vi "cwave_herbert.vi"(5 "Timing input":path=path "D:/Herbert/MeTimingDLL_test/bin/Release/MOTConf.csv", 8 "error in (no error)":errorcluster, 10 "Loop number":i16, 11 "Update rate (kHz)":i32=20) -> (0 "error out":errorcluster)   [LabVIEW 2009]
uses:
  dll.dll
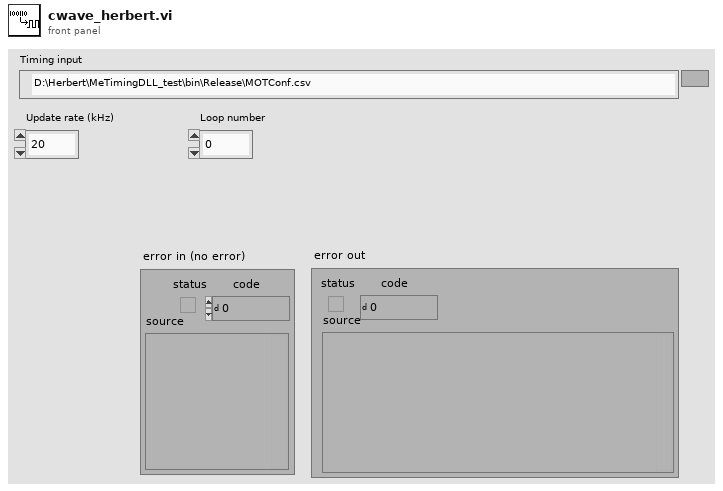
[diagram p1: front panel]
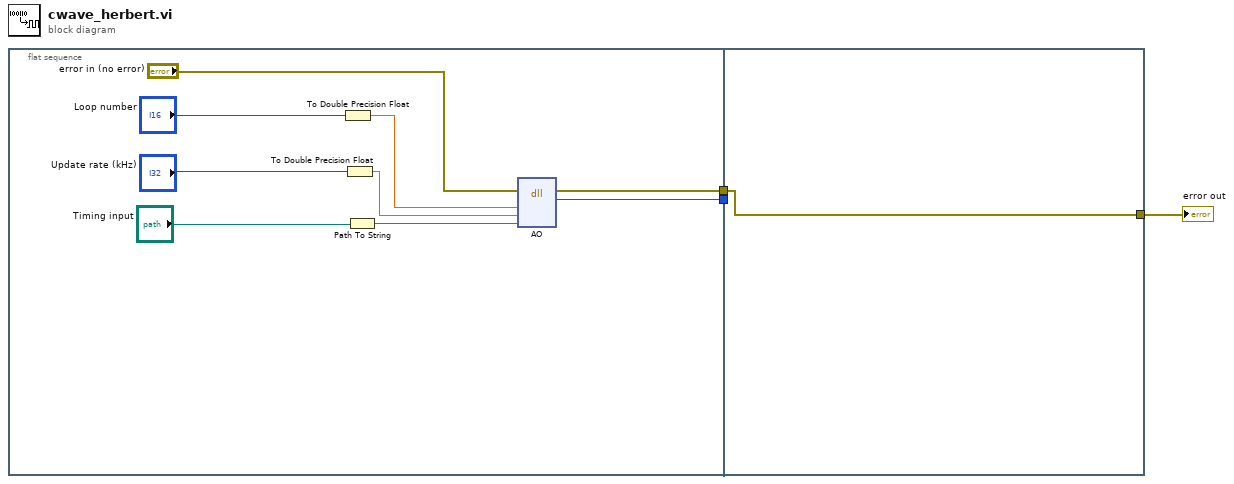
[diagram p0: block diagram]
diagram:
  n1 = flat-sequence {
    tunnel: [w5] -> w3
    tunnel: [w4] -> w2
    tunnel: w3 -> [w13]
    tunnel: w2 -> [_]
    tunnel: [w13] -> w1
    frame #0 {
      n2 = To Double Precision Float(number="Loop number") -> (double precision float=w8:dbl)
      n3 = To Double Precision Float(number="Update rate (kHz)") -> (double precision float=w7:dbl)
      n4 = Path To String(path="Timing input") -> (string=w6:string)
      n5 = dll-call lib="D:/Herbert/MeTimingDLL_test/bin/Release/dll.dll" fn="AO"(error in="error in (no error)", "loop"=w8, "sample_rate"=w7, "conf_path"=w6) -> (error out=w5:errorcluster, "ret"=w4:i32)  [unwired: 5 in, 1 out]
    }
    frame #1 {
    }
  }
  "error out" <- w1
